vi "RIB Req - eSTOP 1 - Normal Operation.vi"(0 "Limits File Path":path, 5 "Results File Path":path, 11 "error in":errorcluster) -> (4 "Results Data Array":string[][](array[string]), 15 "error out":errorcluster)   [LabVIEW 2024]
doc: "Template test"
uses:
  <vilib>/addons/_JKI Toolkits/State Machine/_JKI_lib_State_Machine.llb/Select State(s)_err__jki_lib_state_machine.vi
  <vilib>/addons/_JKI Toolkits/State Machine/_JKI_lib_State_Machine.llb/Periodic Trigger__ogtk__JKI-SM__jki_lib_state_machine.vi
  <userlib>/_OpenG.lib/file/file.llb/Strip Path Extension - String__ogtk.vi
  <vilib>/Utility/file.llb/Read Delimited Spreadsheet (string).vi
  <vilib>/addons/_JKI Toolkits/State Machine/_JKI_lib_State_Machine.llb/Select State(s)_bool__jki_lib_state_machine.vi
  <userlib>/_OpenG.lib/file/file.llb/openg_file.lvlib
  <userlib>/_OpenG.lib/appcontrol/appcontrol.llb/openg_application_control.lvlib
  <userlib>/_OpenG.lib/time/time.llb/openg_time.lvlib
  <vilib>/Utility/file.llb/Write Delimited Spreadsheet (string).vi
panel:
  out "Timeout - Error Test 2":dbl(slide) scale=0.0..3.0
  out "Wait - Reset":u32(slide)=1 scale=0.0..10.0
  in  "eSTOP 1 State Error Test":string
  in  "eSTOP 1 State Test":string
  in  "Read Start":string
  in  "Read Set":string
  out "Timeout - Error Test":dbl(slide) scale=0.0..3.0
  in  "eSTOP 1 Error Test":string
  in  "eSTOP 1 Test":string
  in  "connection ID":refnum<k16>
  in  "handle out":u64
  in  "Exit":bool
  # "eSTOP 1 Test"
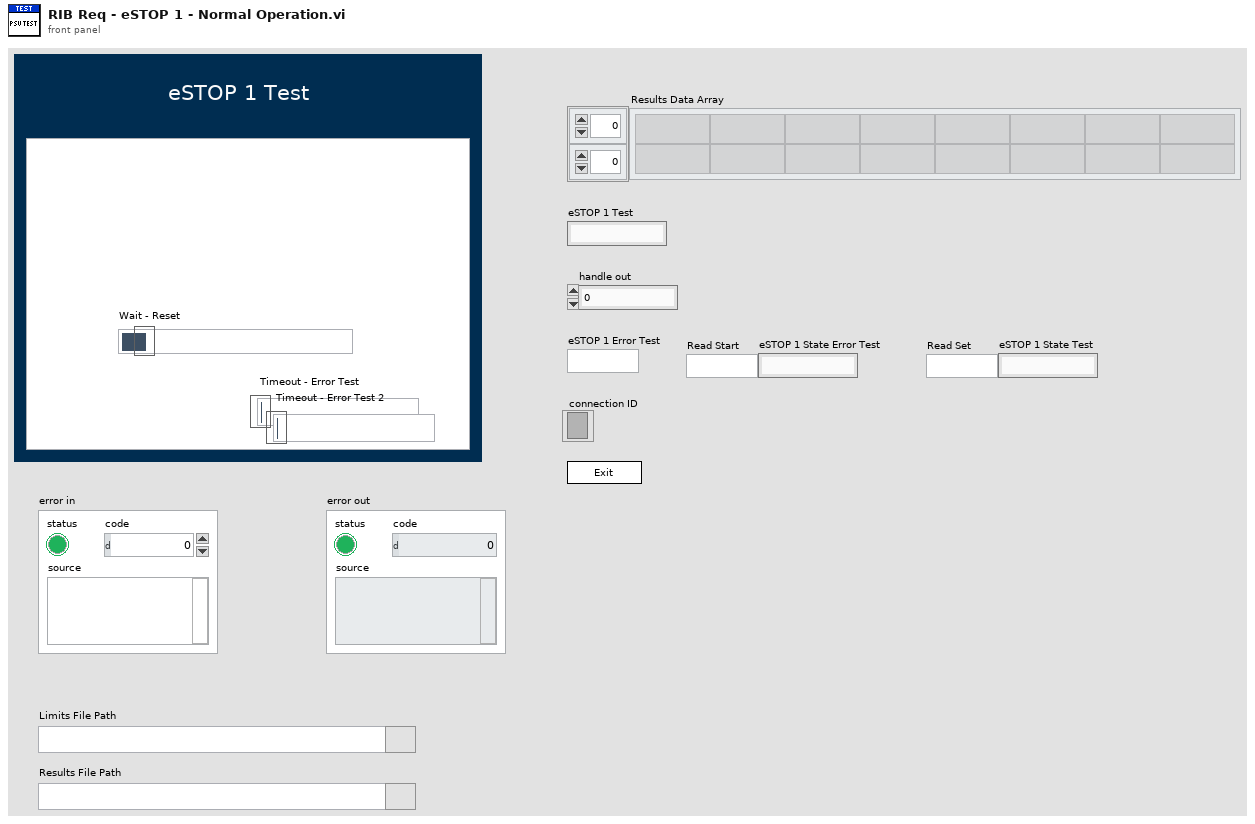
[diagram p1: front panel]
types:
  T1 = enum32{"Invalid", "Standard", "Closed", "Hidden", "Minimized", "Maximized"}
  T2 = enum32{"invalid app kind", "Development System", "Run Time System", "Student Edition", "Embedded LabVIEW", "Evaluation", "Custom"}
  T3 = typedef "FGV - Enum" = enum16{"Cleanup", "Get Data", "Open UDP", "Initialise DAQ", "Initialise I2C"}
  T4 = enum16{"Start Timer", "Get Time", "Pause", "Unpause"}
  T5 = cluster{"Core":cluster{"Current VI Reference":refnum<vi>, "Close Panel on Exit?":bool}, "Limits File Path":path, "Test Limits":string[][], "Results Data Array":string[][], "Results File Path":path, "Voltage":dbl, "connection ID":refnum<k16>, "handle out":u64, "eSTOP 1 Test":string, "eSTOP 1 Error Test":string, "Read Set":string, "Read Start ":string, "eSTOP 1 State Test":string, "eSTOP 1 State Error Test":string}
  T6 = cluster{"Current VI Reference":refnum<vi>, "Close Panel on Exit?":bool}
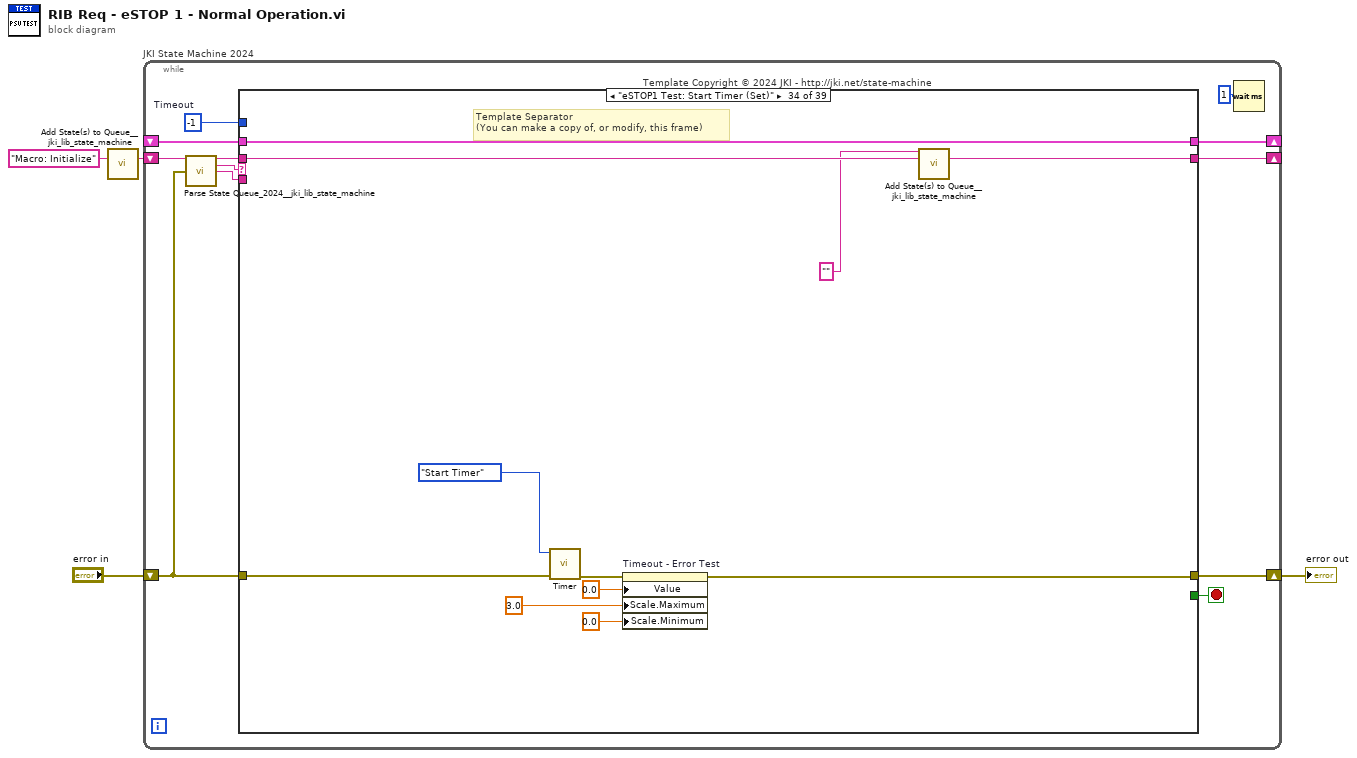
[diagram p0: block diagram]
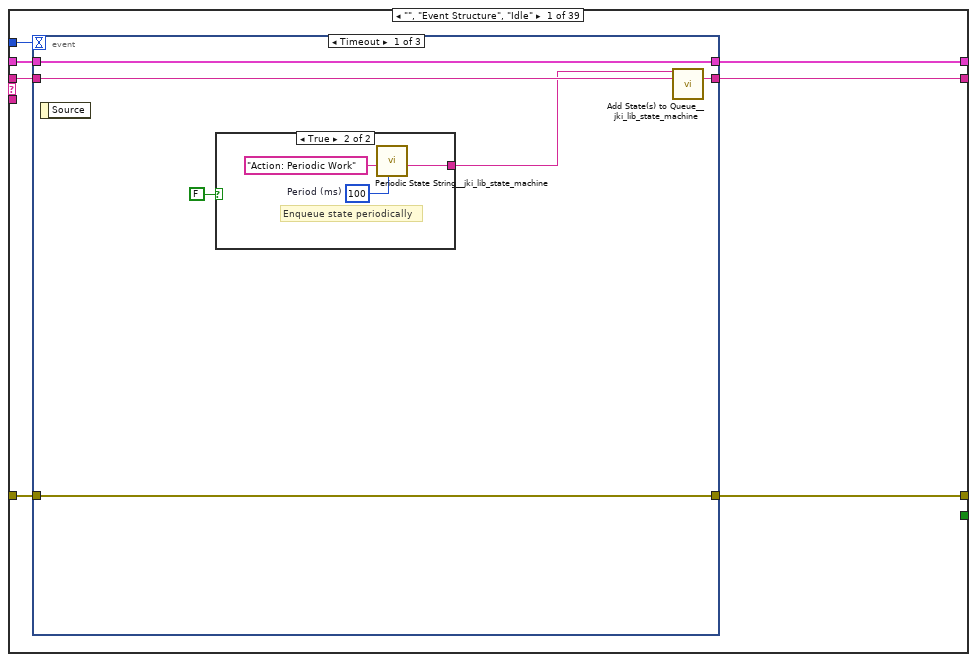
[diagram p2: hidden frame]
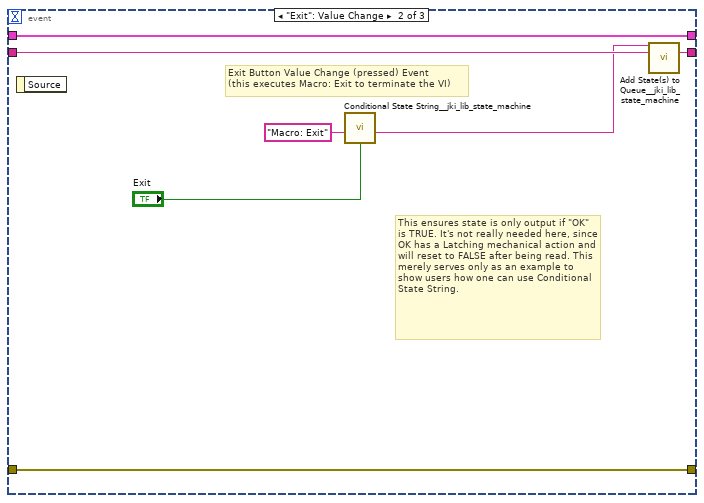
[diagram p4: hidden frame]
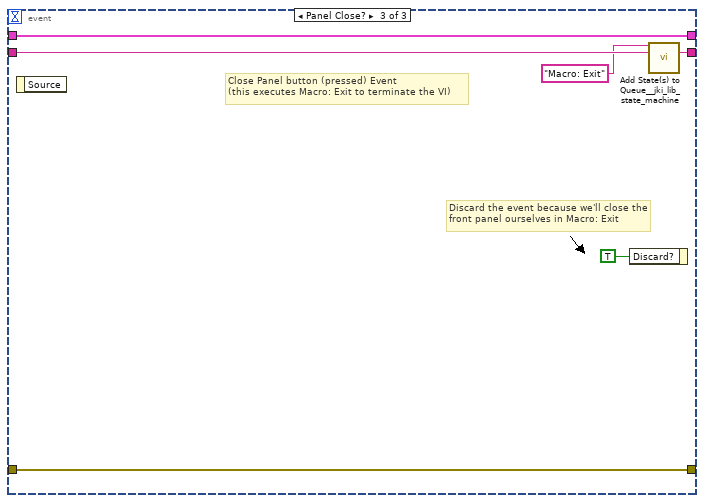
[diagram p5: hidden frame]
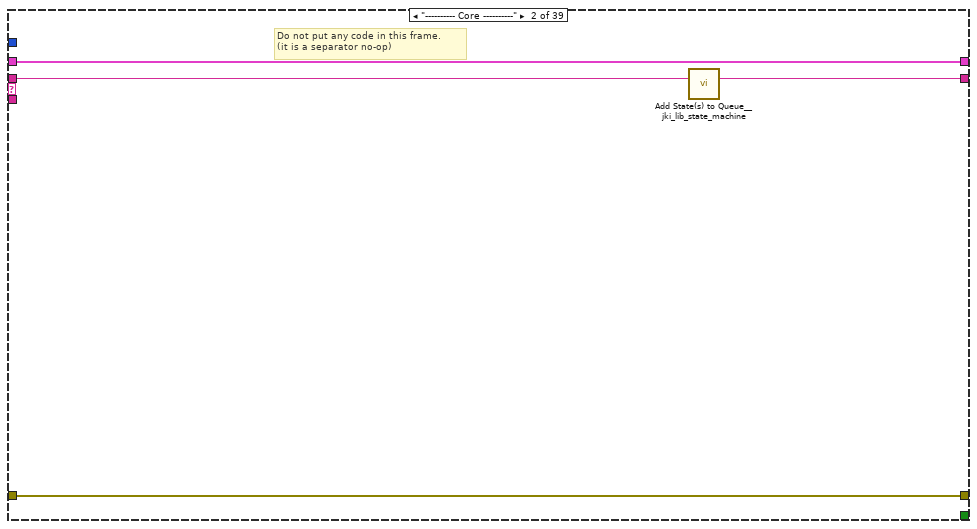
[diagram p6: hidden frame]
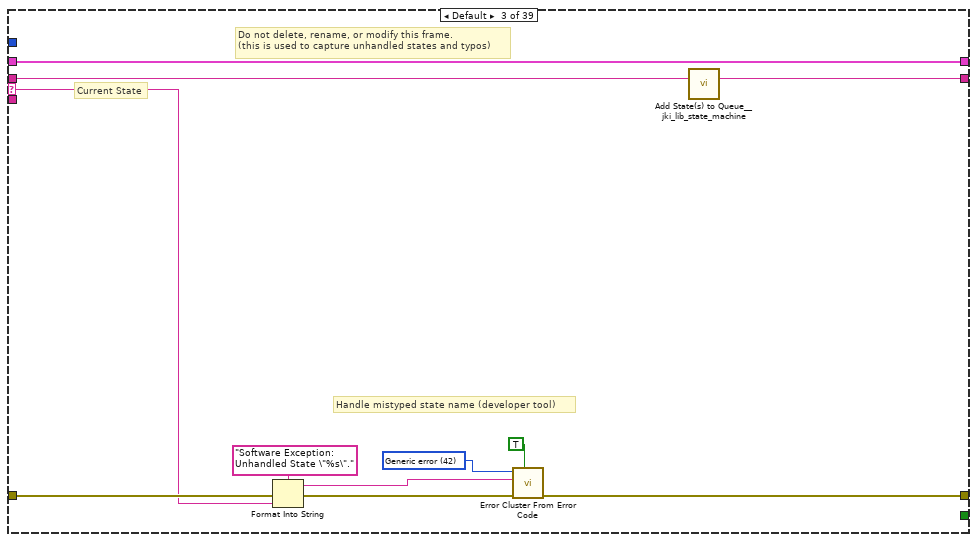
[diagram p7: hidden frame]
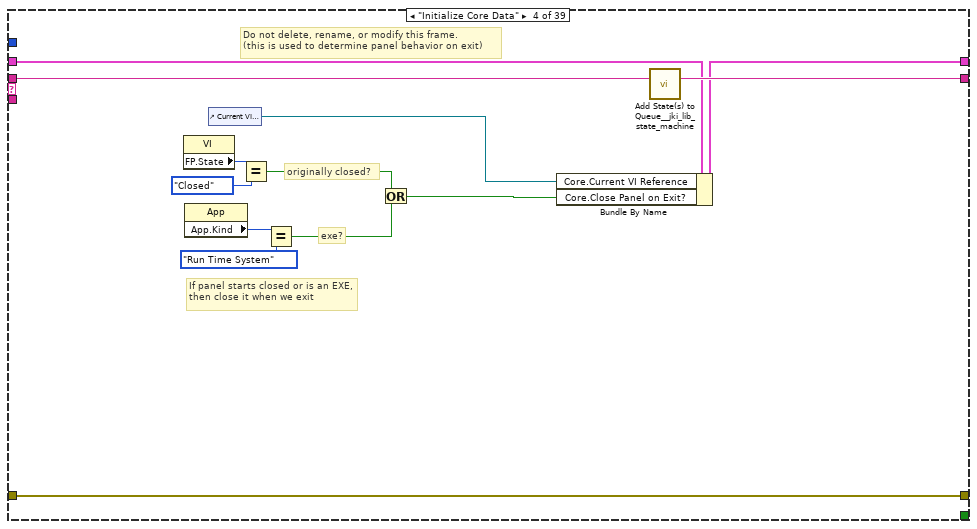
[diagram p8: hidden frame]
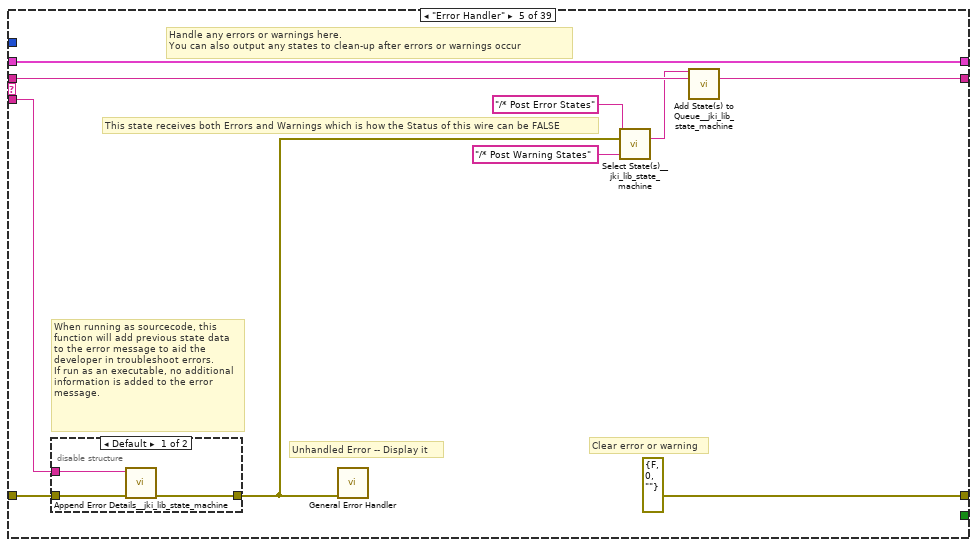
[diagram p9: hidden frame]
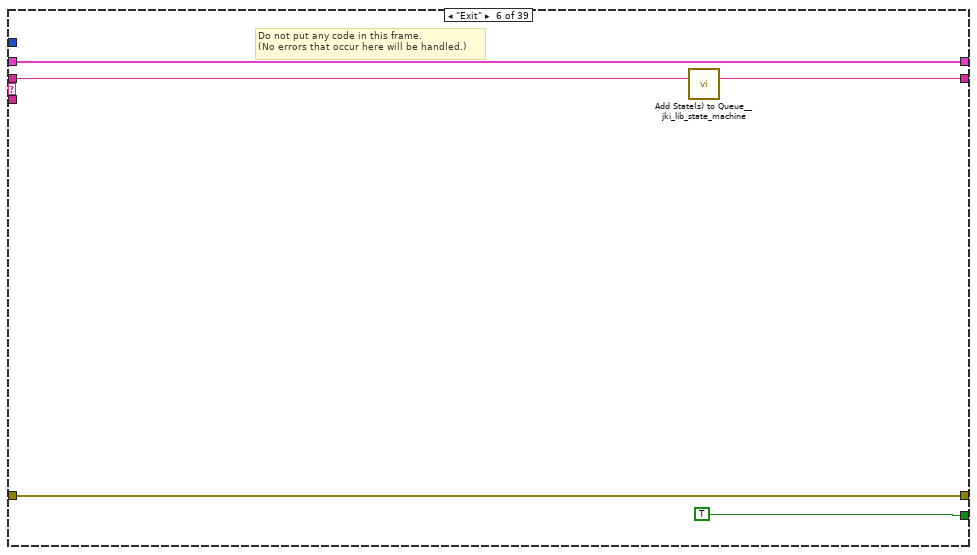
[diagram p11: hidden frame]
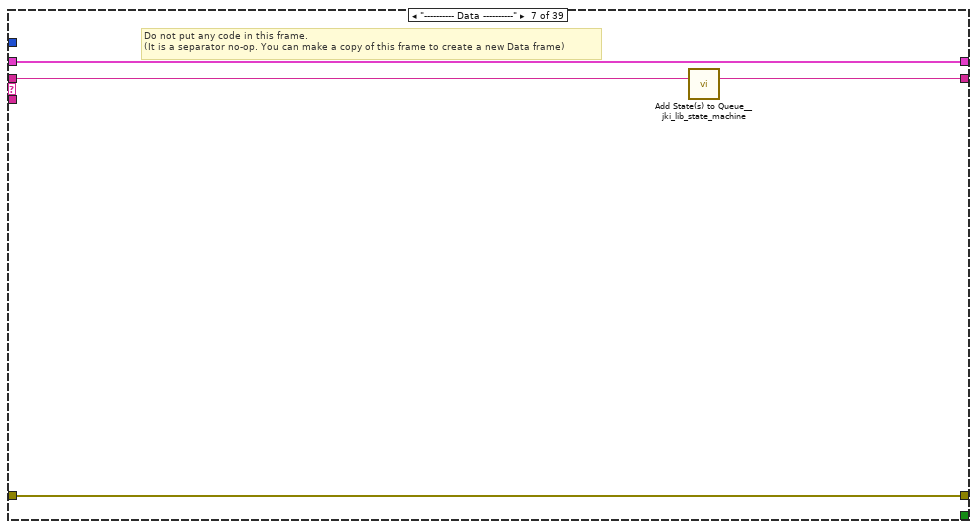
[diagram p12: hidden frame]
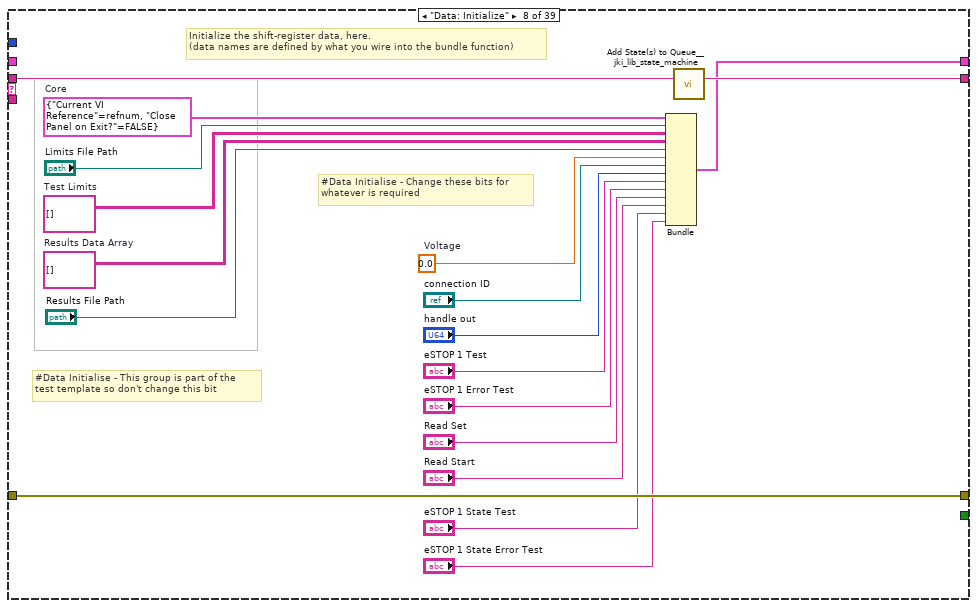
[diagram p13: hidden frame]
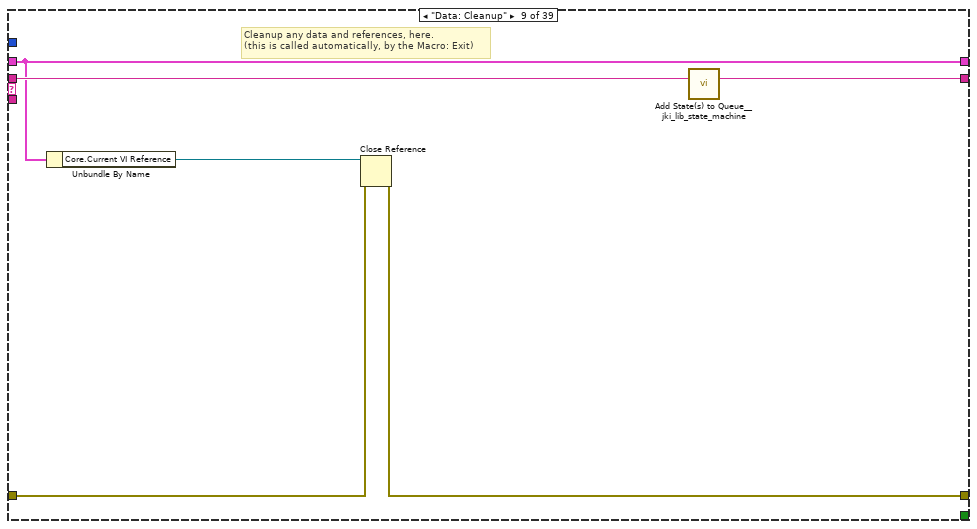
[diagram p14: hidden frame]
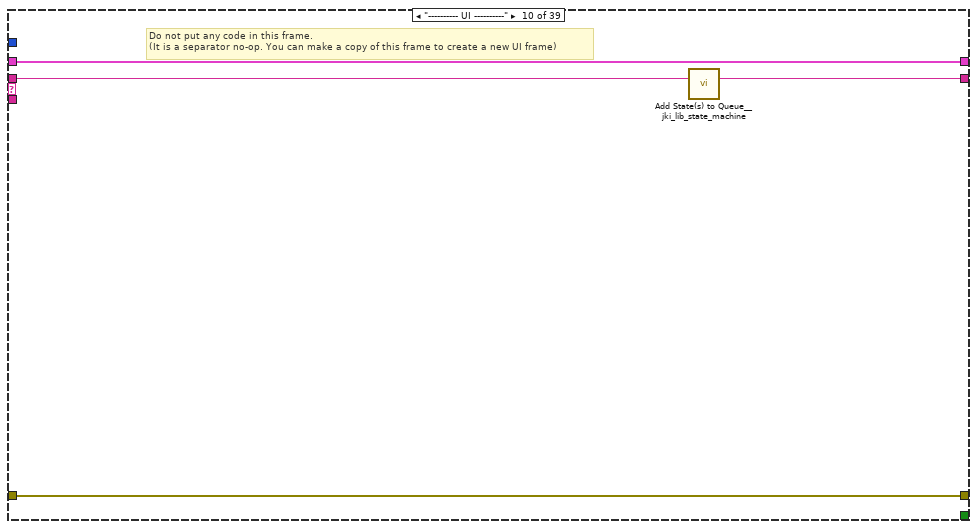
[diagram p15: hidden frame]
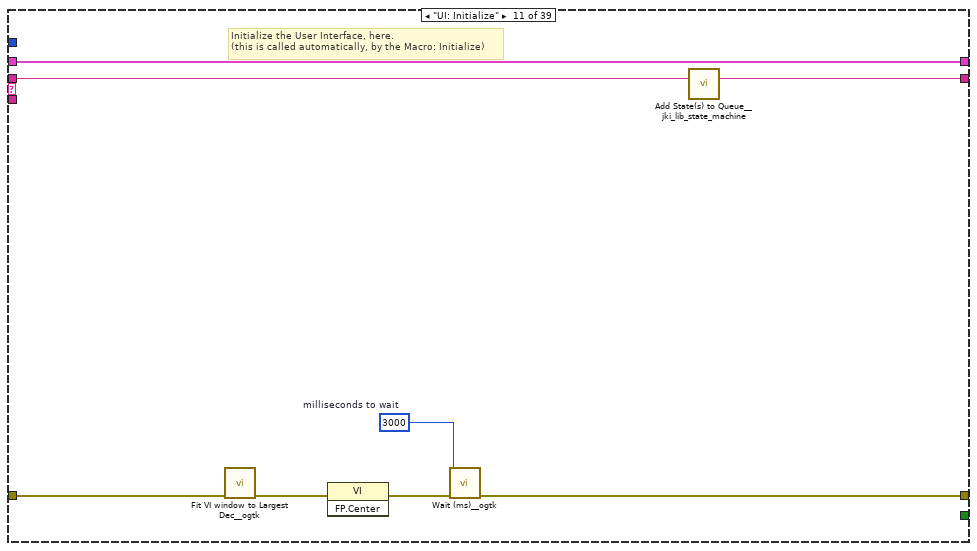
[diagram p16: hidden frame]
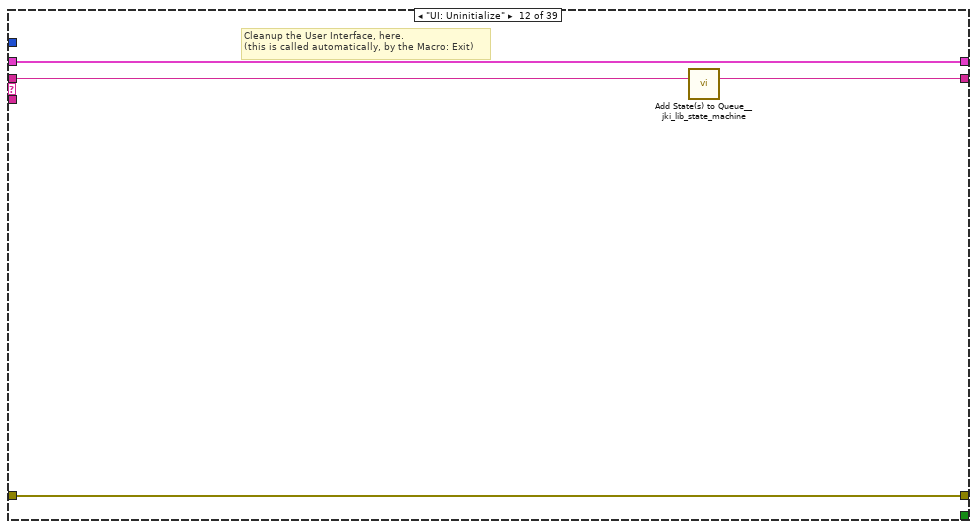
[diagram p17: hidden frame]
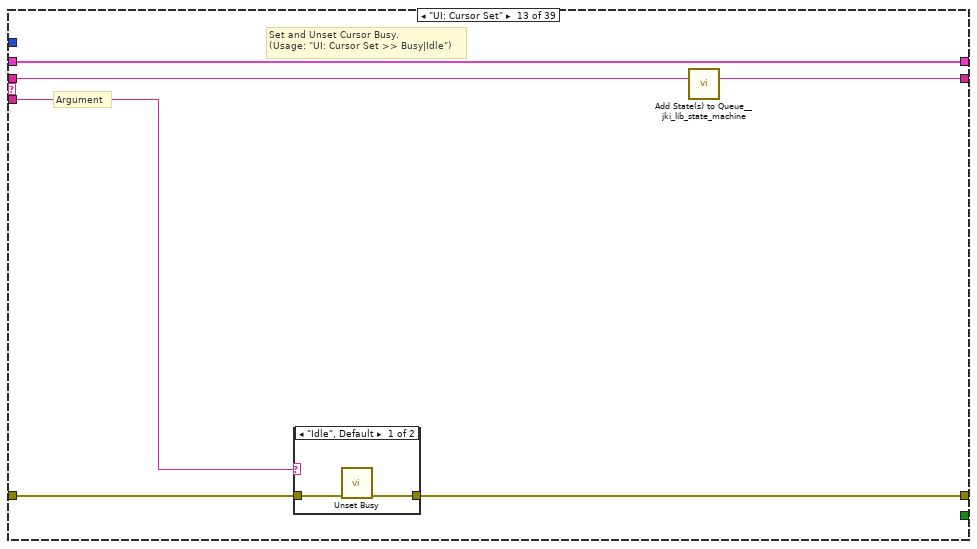
[diagram p18: hidden frame]
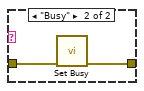
[diagram p19: hidden frame]
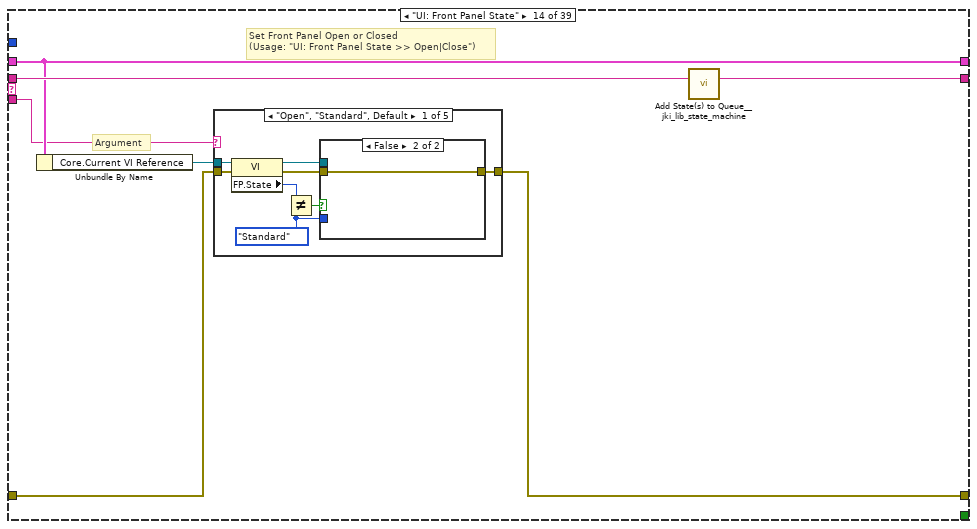
[diagram p20: hidden frame]
diagram:
  n1 = call <vilib>:"Add State(s) to Queue__jki_lib_state_machine.vi"("State(s) in (\"\")"="Macro: Initialize") -> ("States Out"=w4:string)  [unwired: 14 in]
  n2 = while "JKI State Machine 2024" {
    shift-right: [w9] -> _
    shift-left: _ -> [w8]
    shift-right: [w12] -> w1
    shift-left: "error in" -> [w6]
    shift-right: [w11] -> _
    shift-left: w4 -> [w13]
    stop <- w10 stop-if-true
    w7 = -1  # Timeout
    # "Template Copyright © 2024 JKI - http://jki.net/state-machine"
    n3 = call <vilib>:"Parse State Queue_2024__jki_lib_state_machine.vi"("State Queue"=w13, "Error In (no error)"=w6) -> ("Remaining States"=w15:string, "Current State"=w16:string, "Arguments"=w14:string)  [unwired: 11 in]
    n4 = case shown="\"eSTOP1 Test: Start Timer (Set)\"" w16 {
      selector: w16 -> [_ _ w50 _ _ _ _ _ _ _ _ _ _ _ _ _ _ _ _ _ _ _ _ _ _ _ _ _ _ _ _ _ _ _ _ _ _ _ _]
      tunnel: w15 -> [w23 w49 w54 w73 w83 w92 w96 w114 w120 w124 w132 w136 w142 w153 w222 w227 w232 w237 w242 w251 w255 w268 w285 w298 w311 w324 w337 w350 w354 w363 w367 w376 w385 w396 w418 w430 w441 w462 w474]
      tunnel: w14 -> [_ _ _ _ w78 _ _ _ _ _ _ _ w137 w147 _ _ _ _ _ _ _ _ _ _ _ _ _ _ _ _ _ _ _ _ _ _ _ _ _]
      tunnel: w8 -> [w21 w46 w52 w66 w80 w90 w93 _ w115 w121 w130 w134 w140 w149 w219 w224 w229 w234 w239 w249 w252 w258 w277 w290 w303 w316 w329 w342 w351 w359 w364 w374 w378 w394 w415 w428 w439 w459 w472]
      tunnel: [w20 w47 w56 w70 errorcluster {"status"=FALSE, "code"=0, "source"=""} ("error out") w89 w94 w111 w116 w122 w128 w133 w138 w150 w220 w225 w230 w235 w240 w246 w253 w264 w282 w295 w308 w321 w334 w347 w352 w361 w365 w371 w380 w387 w399 w422 w432 w443 w466] -> w12
      tunnel: w6 -> [w17 w47 w55 w70 w79 w89 w94 w111 w117 w122 w129 w133 w139 w151 w220 w225 w230 w235 w240 w246 w253 w263 w281 w294 w307 w320 w333 w346 w352 w360 w365 w372 w379 w388 w414 w423 w433 w458 w467]
      tunnel: [w22 w48 w53 w72 w82 w91 w95 w113 w119 w123 w131 w135 w141 w152 w221 w226 w231 w236 w241 w250 w254 w267 w284 w297 w310 w323 w336 w349 w353 w362 w366 w375 w384 w395 w417 w429 w440 w461 w473] -> w11
      tunnel: [_ _ _ _ _ TRUE _ _ _ _ _ _ _ _ _ _ _ _ _ _ _ _ _ _ _ _ _ _ _ _ _ _ _ _ _ _ _ _ _] -> w10
      tunnel: [w19 w46 w52 w71 w80 w90 w93 w112 w115 w121 w130 w134 w140 w149 w219 w224 w229 w234 w239 w249 w252 w257 w276 w289 w302 w315 w328 w341 w351 w359 w364 w373 w377 w394 w416 w428 w439 w460 w472] -> w9
      tunnel: w7 -> [w18 _ _ _ _ _ _ _ _ _ _ _ _ _ _ _ _ _ _ _ _ _ _ _ _ _ _ _ _ _ _ _ _ _ _ _ _ _ _]
      frame "", "Event Structure", "Idle" {
        n5 = event shown="[0] Timeout" {
          selector: _ -> [_ _ _]
          dyn-events: _ -> [_ _ _]
          timeout: w18 -> [_ _ _]
          tunnel: w23 -> [w29 w39 w45]
          tunnel: [w28 w38 w44] -> w22
          tunnel: w21 -> [w26 w36 w42]
          tunnel: [w27 w37 w43] -> w20
          tunnel: w17 -> [w27 w37 w43]
          tunnel: [w26 w36 w42] -> w19
          event Timeout {
            n6 = event-data() -> ()  [unwired: 1 in, 1 out]
            n7 = case shown="True" FALSE {
              tunnel: [_ w32] -> w25
              frame False {
              }
              frame True {
                w30 = u32 100  # Period (ms)
                # "Enqueue state periodically"
                n8 = call <vilib>:"Periodic State String__jki_lib_state_machine.vi"("Period (ms)"=w30, "State"="Action: Periodic Work") -> ("State Out"=w32:string)  [unwired: 9 in]
              }
            }
            n9 = call <vilib>:"Add State(s) to Queue__jki_lib_state_machine.vi"("State(s) in Front (\"\")"=w25, "State(s) in (\"\")"=w29) -> ("States Out"=w28:string)  [unwired: 13 in]
          }
          event "Exit": Value Change {
            # "This ensures state is only output if \"OK\" is TRUE. It's not really needed here, since OK has a Latching mechanical action and will reset to FALSE after being read. This merely serves only as an example to show users how one can use Conditional State String."
            # "Exit Button Value Change (pressed) Event\n(this executes Macro: Exit to terminate the VI)"
            n10 = event-data() -> ()  [unwired: 1 in, 1 out]
            n11 = call <vilib>:"Conditional State String__jki_lib_state_machine.vi"("Do State(s)?"="Exit", "State"="Macro: Exit") -> ("State Out"=w33:string)  [unwired: 7 in]
            n12 = call <vilib>:"Add State(s) to Queue__jki_lib_state_machine.vi"("State(s) in Front (\"\")"=w33, "State(s) in (\"\")"=w39) -> ("States Out"=w38:string)  [unwired: 13 in]
          }
          event Panel Close? {
            # "Discard the event because we'll close the front panel ourselves in Macro: Exit"
            # "Close Panel button (pressed) Event\n(this executes Macro: Exit to terminate the VI)"
            n13 = event-data() -> ()  [unwired: 1 in, 1 out]
            n14 = event-data("Discard?"=TRUE) -> ()  [unwired: 1 in, 1 out]
            n15 = call <vilib>:"Add State(s) to Queue__jki_lib_state_machine.vi"("State(s) in Front (\"\")"="Macro: Exit", "State(s) in (\"\")"=w45) -> ("States Out"=w44:string)  [unwired: 13 in]
          }
        }
      }
      frame "---------- Core ----------" {
        # "Do not put any code in this frame.\n(it is a separator no-op)"
        n16 = call <vilib>:"Add State(s) to Queue__jki_lib_state_machine.vi"("State(s) in (\"\")"=w49) -> ("States Out"=w48:string)  [unwired: 14 in]
      }
      frame Default {
        w59 = 42 items=["No error", "Argument error", "Memory is full", "Out of zone", "End of file", "File already open", "Generic file I/O error", "File not found", "File permission error", "Disk is full", "Duplicate path", "Too many files open", "System feature not enabled", "Resource file not found", "Cannot add resource", "Resource not found", "Image not found", "Image memory error", "Pen does not exist", "Config type invalid", "Config token not found", "Config parse error", "Config memory error", "Bad external code format", "Bad external code offset", "External code not present", "Null window", "Destroy window error", "Null menu", "Print aborted", "Bad print record", "Print driver error", "Windows error during printing", "Memory error during printing", "Print dialog error", "Generic print error", "Invalid device refnum", "Device not found", "Device parameter error", "Device unit error", "Cannot open device", "Device call aborted", "Generic error", "Cancelled by user", "Object ID too low", "Object ID too high", "Object not in heap", "Unknown heap", "Unknown object (invalid DefProc)", "Unknown object (DefProc not in table)", "Message out of range", "Invalid (null) method", "Unknown message", "Manager call not supported", "Bad address", "Network operation in progress", "Network operation timed out", "Connection is busy", "Network attribute not supported", "Network error", "Address in use", "System out of memory", "Connection aborted", "Connection refused", "Not connected", "Already connected", "Connection closed", "Initialization error (interapplication manager)", "Bad occurrence", "Wait on unbound occurrence handler", "Occurrence queue overflow", "Datalog type conflict", "Unused", "Unrecognized type (interapplication manager)", "Memory corrupt", "Failed to make temporary DLL", "Old CIN version", "Drag socket not found", "Failed to load drop-object", "Failed to register OLE object", "Failed to release OLE object", "Format specifier type mismatch", "Unknown format specifier", "Too few format specifiers", "Too many format specifiers", "Scan failed", "Newer CIN version", "Error converting to variant", "Runtime menu error", "Password tampered", "Variant attribute not found", "Incompatible variant data type", "Event data is not available", "Event Store is not present", "Occurrence is not found", "Event Queue is not created", "Event info is not available", "Refnum passed is NULL", "Error retrieving Class GUID", "Error retrieving CoClass GUID", "Error retrieving TypeLib GUID.", "Bad built application magic bytes.", "Specific driver is different from the specific driver associated with the Logical Name.", "There is no session opened to the class driver.", "Max Error", "MAX - Error with config objects", "MAX - Error loading configuration", "MAX - Group not supported"]
        # "Current State"
        # "Do not delete, rename, or modify this frame.\n(this is used to capture unhandled states and typos)"
        # "Handle mistyped state name (developer tool)"
        n17 = Format Into String(format string="Software Exception: Unhandled State \"%s\"." ("message"), error in=w55, w50) -> (resulting string=w58:string, error out=w57:errorcluster)  [unwired: 1 in]
        n18 = call <vilib>:"Error Cluster From Error Code.vi"("show call chain? (False)"=TRUE, "error in (no error)"=w57, "error message (\"\")"=w58, "error code (0)"=w59) -> ("error out"=w56:errorcluster)  [unwired: 5 in]
        n19 = call <vilib>:"Add State(s) to Queue__jki_lib_state_machine.vi"("State(s) in (\"\")"=w54) -> ("States Out"=w53:string)  [unwired: 14 in]
      }
      frame "Initialize Core Data" {
        # "Do not delete, rename, or modify this frame.\n(this is used to determine panel behavior on exit)"
        # "originally closed?"
        # "exe?"
        # "If panel starts closed or is an EXE, then close it when we exit"
        n20 = property class="VI"() -> ("FP.State"=w63:T1)  [unwired: 2 in, 2 out]
        n21 = property class="App"() -> ("App.Kind"=w69:T2)  [unwired: 2 in, 2 out]
        n22 = control-ref of="Current VI Reference"() -> (w64:refnum<vi>)
        n23 = Equal?(x=w63, y=T1."Closed" ("Front Panel Window:State")) -> (x = y?=w61:bool)
        n24 = Equal?(x=w69, y=T2."Run Time System" ("Application:Kind")) -> (x = y?=w67:bool)
        n25 = Or(x=w61, y=w67) -> (x .or. y?=w65:bool)
        n26 = Bundle By Name(cluster=w66, "Core.Current VI Reference"=w64, "Core.Close Panel on Exit?"=w65) -> (w71:T5)
        n27 = call <vilib>:"Add State(s) to Queue__jki_lib_state_machine.vi"("State(s) in (\"\")"=w73) -> ("States Out"=w72:string)  [unwired: 14 in]
      }
      frame "Error Handler" {
        # "When running as sourcecode, this function will add previous state data to the error message to aid the developer in troubleshoot errors.\nIf run as an executable, no additional information is added to the error message."
        # "This state receives both Errors and Warnings which is how the Status of this wire can be FALSE"
        # "Unhandled Error -- Display it"
        # "Handle any errors or warnings here.\nYou can also output any states to clean-up after errors or warnings occur"
        # "Clear error or warning"
        n28 = disable-structure shown="Default" {
          disable-tunnel: w79 -> [w86 w87]
          disable-tunnel: w78 -> [w85 _]
          disable-tunnel: [w84 w87] -> w77
          frame condition #0 (active) {
            n29 = call <vilib>:"Append Error Details__jki_lib_state_machine.vi"("error in (no error)"=w86, "Previous State and Argument(s)"=w85) -> ("error out"=w84:errorcluster)  [unwired: 9 in]
          }
          frame condition #1 {
          }
        }
        n30 = call <vilib>:"General Error Handler.vi"("error in (no error)"=w77) -> ()  [unwired: 10 in, 5 out]
        n31 = call-poly <vilib>:"Select State(s)__jki_lib_state_machine.vi"("State(s) if True (\"\")"="/* Post Error States", "Select"=w77, "State(s) if False (\"\")"="/* Post Warning States") -> ("States Out"=w75:string)  [unwired: 12 in]
        n32 = call <vilib>:"Add State(s) to Queue__jki_lib_state_machine.vi"("State(s) in Front (\"\")"=w75, "State(s) in (\"\")"=w83) -> ("States Out"=w82:string)  [unwired: 13 in]
      }
      frame "Exit" {
        # "Do not put any code in this frame.\n(No errors that occur here will be handled.)"
        n33 = call <vilib>:"Add State(s) to Queue__jki_lib_state_machine.vi"("State(s) in (\"\")"=w92) -> ("States Out"=w91:string)  [unwired: 14 in]
      }
      frame "---------- Data ----------" {
        # "Do not put any code in this frame.\n(It is a separator no-op. You can make a copy of this frame to create a new Data frame)"
        n34 = call <vilib>:"Add State(s) to Queue__jki_lib_state_machine.vi"("State(s) in (\"\")"=w96) -> ("States Out"=w95:string)  [unwired: 14 in]
      }
      frame "Data: Initialize" {
        w105 = 0.0  # Voltage
        w107 = string[][] []  # Results Data Array
        w108 = string[][] []  # Test Limits
        w110 = T6 {"Current VI Reference"=refnum, "Close Panel on Exit?"=FALSE}  # Core
        # "#Data Initialise - Change these bits for\nwhatever is required"
        # "#Data Initialise - This group is part of the\ntest template so don't change this bit"
        # "Initialize the shift-register data, here.\n(data names are defined by what you wire into the bundle function)"
        n35 = Bundle("Core"=w110, "Limits File Path"="Limits File Path", "Test Limits"=w108, "Results Data Array"=w107, "Results File Path"="Results File Path", "Voltage"=w105, "connection ID"="connection ID", "handle out"="handle out", "eSTOP 1 Test"="eSTOP 1 Test", "eSTOP 1 Error Test"="eSTOP 1 Error Test", "Read Set"="Read Set", "Read Start"="Read Start", "eSTOP 1 State Test"="eSTOP 1 State Test", "eSTOP 1 State Error Test"="eSTOP 1 State Error Test") -> (w112:T5)  [unwired: 1 in]
        n36 = call <vilib>:"Add State(s) to Queue__jki_lib_state_machine.vi"("State(s) in (\"\")"=w114) -> ("States Out"=w113:string)  [unwired: 14 in]
      }
      frame "Data: Cleanup" {
        # "Cleanup any data and references, here.\n(this is called automatically, by the Macro: Exit)"
        n37 = Unbundle By Name(w115) -> ("Core.Current VI Reference"=w118:refnum<vi>)
        n38 = Close Reference(reference=w118, error in (no error)=w117) -> (error out=w116:errorcluster)
        n39 = call <vilib>:"Add State(s) to Queue__jki_lib_state_machine.vi"("State(s) in (\"\")"=w120) -> ("States Out"=w119:string)  [unwired: 14 in]
      }
      frame "---------- UI ----------" {
        # "Do not put any code in this frame.\n(It is a separator no-op. You can make a copy of this frame to create a new UI frame)"
        n40 = call <vilib>:"Add State(s) to Queue__jki_lib_state_machine.vi"("State(s) in (\"\")"=w124) -> ("States Out"=w123:string)  [unwired: 14 in]
      }
      frame "UI: Initialize" {
        w127 = u32 3000  # milliseconds to wait
        # "Initialize the User Interface, here.\n(this is called automatically, by the Macro: Initialize)"
        n41 = call <userlib>:"Fit VI window to Largest Dec__ogtk.vi"("error in (no error)"=w129) -> ("error out"=w125:errorcluster)  [unwired: 5 in, 1 out]
        n42 = invoke class="VI" method="FP.Center"(error in=w125) -> (error out=w126:errorcluster)  [unwired: 2 in, 2 out]
        n43 = call <userlib>:"Wait (ms)__ogtk.vi"("error in (no error)"=w126, "milliseconds to wait"=w127) -> ("error out"=w128:errorcluster)  [unwired: 8 in, 1 out]
        n44 = call <vilib>:"Add State(s) to Queue__jki_lib_state_machine.vi"("State(s) in (\"\")"=w132) -> ("States Out"=w131:string)  [unwired: 14 in]
      }
      frame "UI: Uninitialize" {
        # "Cleanup the User Interface, here.\n(this is called automatically, by the Macro: Exit)"
        n45 = call <vilib>:"Add State(s) to Queue__jki_lib_state_machine.vi"("State(s) in (\"\")"=w136) -> ("States Out"=w135:string)  [unwired: 14 in]
      }
      frame "UI: Cursor Set" {
        # "Argument"
        # "Set and Unset Cursor Busy.\n(Usage: \"UI: Cursor Set >> Busy|Idle\")"
        n46 = case shown="\"Idle\", Default" w137 {
          tunnel: w139 -> [w144 w146]
          tunnel: [w143 w145] -> w138
          frame "Idle", Default {
            n47 = call <vilib>:"Unset Busy.vi"("error in (no error)"=w144) -> ("error out"=w143:errorcluster)  [unwired: 10 in]
          }
          frame "Busy" {
            n48 = call <vilib>:"Set Busy.vi"("error in (no error)"=w146) -> ("error out"=w145:errorcluster)  [unwired: 9 in, 1 out]
          }
        }
        n49 = call <vilib>:"Add State(s) to Queue__jki_lib_state_machine.vi"("State(s) in (\"\")"=w142) -> ("States Out"=w141:string)  [unwired: 14 in]
      }
      frame "UI: Front Panel State" {
        # "Argument"
        # "Set Front Panel Open or Closed\n(Usage: \"UI: Front Panel State >> Open|Close\")"
        n50 = Unbundle By Name(w149) -> ("Core.Current VI Reference"=w148:refnum<vi>)
        n51 = case shown="\"Open\", \"Standard\", Default" w147 {
          tunnel: w151 -> [w159 w174 w185 w198 w211]
          tunnel: [w161 w175 w187 w200 w213] -> w150
          tunnel: w148 -> [w160 w172 w186 w199 w212]
          frame "Open", "Standard", Default {
            w154 = T1."Standard" ("State")
            n52 = property class="VI"(reference=w160, error in=w159) -> (reference out=w157:refnum<vi>, error out=w158:errorcluster, "FP.State"=w156:T1)
            n53 = Not Equal?(x=w156, y=w154) -> (x != y?=w155:bool)
            n54 = case shown="False" w155 {
              tunnel: [w165 w167] -> w161
              tunnel: w158 -> [w164 w167]
              tunnel: w157 -> [w163 _]
              tunnel: w154 -> [w162 _]
              frame True {
                n55 = invoke class="VI" method="FP.Open"(reference=w163, error in=w164, "Activate"=TRUE, "State"=w162) -> (error out=w165:errorcluster)  [unwired: 1 in, 4 out]
              }
              frame False {
              }
            }
          }
          frame "Close", "Closed" {
            n56 = property class="VI"(reference=w172, error in=w174) -> (reference out=w171:refnum<vi>, error out=w173:errorcluster, "FP.State"=w169:T1)
            n57 = Not Equal?(x=w169, y=T1."Closed" ("Front Panel Window:State")) -> (x != y?=w168:bool)
            n58 = case shown="True" w168 {
              tunnel: [w176 w179] -> w175
              tunnel: w173 -> [w176 w178]
              tunnel: w171 -> [_ w177]
              frame False {
              }
              frame True {
                n59 = invoke class="VI" method="FP.Close"(reference=w177, error in=w178) -> (error out=w179:errorcluster)  [unwired: 1 in, 2 out]
              }
            }
          }
          frame "Hidden", "Hide" {
            w180 = T1."Hidden" ("State")
            n60 = property class="VI"(reference=w186, error in=w185) -> (reference out=w183:refnum<vi>, error out=w184:errorcluster, "FP.State"=w182:T1)
            n61 = Not Equal?(x=w182, y=w180) -> (x != y?=w181:bool)
            n62 = case shown="True" w181 {
              tunnel: [w191 w192] -> w187
              tunnel: w184 -> [w190 w192]
              tunnel: w183 -> [w189 _]
              tunnel: w180 -> [w188 _]
              frame True {
                n63 = invoke class="VI" method="FP.Open"(reference=w189, error in=w190, "State"=w188) -> (error out=w191:errorcluster)  [unwired: 2 in, 4 out]
              }
              frame False {
              }
            }
          }
          frame "Minimize", "Minimized" {
            w193 = T1."Minimized" ("State")
            n64 = property class="VI"(reference=w199, error in=w198) -> (reference out=w196:refnum<vi>, error out=w197:errorcluster, "FP.State"=w195:T1)
            n65 = Not Equal?(x=w195, y=w193) -> (x != y?=w194:bool)
            n66 = case shown="True" w194 {
              tunnel: [w204 w205] -> w200
              tunnel: w197 -> [w203 w205]
              tunnel: w196 -> [w202 _]
              tunnel: w193 -> [w201 _]
              frame True {
                n67 = invoke class="VI" method="FP.Open"(reference=w202, error in=w203, "State"=w201) -> (error out=w204:errorcluster)  [unwired: 2 in, 4 out]
              }
              frame False {
              }
            }
          }
          frame "Maximize", "Maximized" {
            w206 = T1."Maximized" ("State")
            n68 = property class="VI"(reference=w212, error in=w211) -> (reference out=w209:refnum<vi>, error out=w210:errorcluster, "FP.State"=w208:T1)
            n69 = Not Equal?(x=w208, y=w206) -> (x != y?=w207:bool)
            n70 = case shown="True" w207 {
              tunnel: [w217 w218] -> w213
              tunnel: w210 -> [w216 w218]
              tunnel: w209 -> [w215 _]
              tunnel: w206 -> [w214 _]
              frame True {
                n71 = invoke class="VI" method="FP.Open"(reference=w215, error in=w216, "State"=w214) -> (error out=w217:errorcluster)  [unwired: 2 in, 4 out]
              }
              frame False {
              }
            }
          }
        }
        n72 = call <vilib>:"Add State(s) to Queue__jki_lib_state_machine.vi"("State(s) in (\"\")"=w153) -> ("States Out"=w152:string)  [unwired: 14 in]
      }
      frame "---------- Macro ----------" {
        # "Do not put any code in this frame.\n(It is a separator no-op. You can make a copy of this frame to create a new Macro frame)"
        n73 = call <vilib>:"Add State(s) to Queue__jki_lib_state_machine.vi"("State(s) in (\"\")"=w222) -> ("States Out"=w221:string)  [unwired: 14 in]
      }
      frame "Macro: Initialize" {
        # "Initialization Macro\n(This is called once, when the VI starts)"
        n74 = call <vilib>:"Add State(s) to Queue__jki_lib_state_machine.vi"("State(s) in Front (\"\")"="Data: Initialize\nInitialize Core Data\nUI: Initialize\nUI: Front Panel State >> Open\neSTOP1 Test: Initialise\nMacro: Test", "State(s) in (\"\")"=w227) -> ("States Out"=w226:string)  [unwired: 13 in]
      }
      frame "Macro: Test" {
        # "#Test Macro - Add the sequence \nfor measurments and limits testing here"
        n75 = call <vilib>:"Add State(s) to Queue__jki_lib_state_machine.vi"("State(s) in Front (\"\")"="Limits Test: Read Limits File\neSTOP1 Test: Initialise", "State(s) in (\"\")"=w232) -> ("States Out"=w231:string)  [unwired: 13 in]
      }
      frame "Macro: Test (Error)" {
        # "#Test Macro - Add the sequence \nfor measurments and limits testing here"
        n76 = call <vilib>:"Add State(s) to Queue__jki_lib_state_machine.vi"("State(s) in Front (\"\")"="eSTOP1 Test: Reset", "State(s) in (\"\")"=w237) -> ("States Out"=w236:string)  [unwired: 13 in]
      }
      frame "Macro: Limits" {
        # "Do not put any code in this frame.\n(It is a separator no-op. You can make a copy of this frame to create a new Macro frame)"
        n77 = call <vilib>:"Add State(s) to Queue__jki_lib_state_machine.vi"("State(s) in Front (\"\")"="Limits Test: eSTOP 1 Test\nLimits Test: eSTOP 1 Error Test\nLimits Test: Read Set\nLimits Test: Read Start\nLimits Test: eSTOP 1 State Error Test\nLimits Test: eSTOP 1 State Test\nResults Data: Write Results Data\nMacro: Exit", "State(s) in (\"\")"=w242) -> ("States Out"=w241:string)  [unwired: 13 in]
      }
      frame "Macro: Exit" {
        # "Exit Macro\n(This is called once, when the VI exits)"
        n78 = Unbundle By Name(w249) -> ("Core.Close Panel on Exit?"=w244:bool)
        n79 = call <vilib>:"Conditional State String__jki_lib_state_machine.vi"("Do State(s)?"=w244, "State"="UI: Front Panel State >> Close") -> ("State Out"=w243:string)  [unwired: 7 in]
        n80 = call <vilib>:"Add State(s) to Queue__jki_lib_state_machine.vi"("State(s) in (\"\")"=w243, "State(s) at Back (\"\")"="UI: Uninitialize\nData: Cleanup\nExit") -> ("States Out"=w247:string)  [unwired: 13 in]
        n81 = call <vilib>:"Add State(s) to Queue__jki_lib_state_machine.vi"("State(s) in Front (\"\")"=w247, "State(s) in (\"\")"=w251) -> ("States Out"=w250:string)  [unwired: 13 in]
      }
      frame "---------- Limits Test ----------" {
        # "Template Separator\n(You can make a copy of, or modify, this frame)"
        n82 = call <vilib>:"Add State(s) to Queue__jki_lib_state_machine.vi"("State(s) in (\"\")"=w255) -> ("States Out"=w254:string)  [unwired: 14 in]
      }
      frame "Limits Test: Read Limits File" {
        w261 = ","  # delimiter (\t)
        n83 = Unbundle By Name(w258) -> ("Limits File Path"=w262:path)
        n84 = Current VI's Path "Test Case Path"() -> (path=w266:path)
        n85 = call-poly <vilib>:"Read Delimited Spreadsheet.vi"("file path (dialog if empty)"=w262, "error in (no error)"=w263, "delimiter (\\t)"=w261) -> ("all rows"=w259:string[][], "error out"=w264:errorcluster)  [unwired: 7 in, 4 out]
        n86 = Strip Path(path=w266) -> (name=w265:string)  [unwired: 1 out]
        n87 = call-poly <userlib>:"Strip Path Extension__ogtk.vi"("path"=w265) -> ("root"=w260:string)  [unwired: 1 out]
        n88 = for {
          tunnel: w260 -> [w272]
          tunnel: w259 -> [w270] mode=indexing
          tunnel: [w270] -> w256 mode=indexing if=w269
          n89 = Index Array(array=w270) -> (element=w271:string)  [unwired: 1 in]
          n90 = Equal?(x=w272, y=w271) -> (x = y?=w269:bool)
        }
        n91 = Bundle By Name(cluster=w258, "Test Limits"=w256) -> (w257:T5)
        n92 = call <vilib>:"Add State(s) to Queue__jki_lib_state_machine.vi"("State(s) in (\"\")"=w268) -> ("States Out"=w267:string)  [unwired: 14 in]
      }
      frame "Limits Test: eSTOP 1 Test" {
        w278 = "eSTOP 1 Test"  # Sub Test Name
        # "Equal to F1?"
        # "#Limits Testing - Add the sub test name for\ntest included in limits file"
        n93 = Unbundle By Name(w277) -> ("Test Limits"=w279:string[][], "eSTOP 1 Test"=w283:string)
        n94 = Unbundle By Name(w277) -> ("Results Data Array"=w275:string[][])
        n95 = To Variant(anything=w283) -> (Variant=w280:variant)
        n96 = call "Process Results.vi"("error in (no error)"=w281, "Measurement"=w280, "Test Limits"=w279, "Sub Test Name"=w278) -> ("error out"=w282:errorcluster, "Results Data"=w274:string[])  [unwired: 6 in]
        n97 = Build Array (concatenate)(w275, w274) -> (w273:string[][])
        n98 = Bundle By Name(cluster=w277, "Results Data Array"=w273) -> (w276:T5)
        n99 = call <vilib>:"Add State(s) to Queue__jki_lib_state_machine.vi"("State(s) in (\"\")"=w285) -> ("States Out"=w284:string)  [unwired: 14 in]
      }
      frame "Limits Test: eSTOP 1 State Test" {
        w291 = "eSTOP 1 State Test"  # Sub Test Name
        # "Equal to F1?"
        # "#Limits Testing - Add the sub test name for\ntest included in limits file"
        n100 = Unbundle By Name(w290) -> ("Test Limits"=w292:string[][], "eSTOP 1 State Test"=w296:string)
        n101 = Unbundle By Name(w290) -> ("Results Data Array"=w288:string[][])
        n102 = To Variant(anything=w296) -> (Variant=w293:variant)
        n103 = call "Process Results.vi"("error in (no error)"=w294, "Measurement"=w293, "Test Limits"=w292, "Sub Test Name"=w291) -> ("error out"=w295:errorcluster, "Results Data"=w287:string[])  [unwired: 6 in]
        n104 = Build Array (concatenate)(w288, w287) -> (w286:string[][])
        n105 = Bundle By Name(cluster=w290, "Results Data Array"=w286) -> (w289:T5)
        n106 = call <vilib>:"Add State(s) to Queue__jki_lib_state_machine.vi"("State(s) in (\"\")"=w298) -> ("States Out"=w297:string)  [unwired: 14 in]
      }
      frame "Limits Test: Read Set" {
        w304 = "Read Set Test"  # Sub Test Name
        # "Equal to F1?"
        # "#Limits Testing - Add the sub test name for\ntest included in limits file"
        n107 = Unbundle By Name(w303) -> ("Results Data Array"=w301:string[][])
        n108 = Unbundle By Name(w303) -> ("Test Limits"=w305:string[][], "Read Set"=w309:string)
        n109 = To Variant(anything=w309) -> (Variant=w306:variant)
        n110 = call "Process Results.vi"("error in (no error)"=w307, "Measurement"=w306, "Test Limits"=w305, "Sub Test Name"=w304) -> ("error out"=w308:errorcluster, "Results Data"=w300:string[])  [unwired: 6 in]
        n111 = Build Array (concatenate)(w301, w300) -> (w299:string[][])
        n112 = Bundle By Name(cluster=w303, "Results Data Array"=w299) -> (w302:T5)
        n113 = call <vilib>:"Add State(s) to Queue__jki_lib_state_machine.vi"("State(s) in (\"\")"=w311) -> ("States Out"=w310:string)  [unwired: 14 in]
      }
      frame "Limits Test: Read Start" {
        w317 = "Read Start Test"  # Sub Test Name
        # "Equal to F1?"
        # "#Limits Testing - Add the sub test name for\ntest included in limits file"
        n114 = Unbundle By Name(w316) -> ("Results Data Array"=w314:string[][])
        n115 = Unbundle By Name(w316) -> ("Test Limits"=w318:string[][], "Read Start"=w322:string)
        n116 = To Variant(anything=w322) -> (Variant=w319:variant)
        n117 = call "Process Results.vi"("error in (no error)"=w320, "Measurement"=w319, "Test Limits"=w318, "Sub Test Name"=w317) -> ("error out"=w321:errorcluster, "Results Data"=w313:string[])  [unwired: 6 in]
        n118 = Build Array (concatenate)(w314, w313) -> (w312:string[][])
        n119 = Bundle By Name(cluster=w316, "Results Data Array"=w312) -> (w315:T5)
        n120 = call <vilib>:"Add State(s) to Queue__jki_lib_state_machine.vi"("State(s) in (\"\")"=w324) -> ("States Out"=w323:string)  [unwired: 14 in]
      }
      frame "Limits Test: eSTOP 1 Error Test" {
        w330 = "eSTOP 1 Error Test"  # Sub Test Name
        # "Equal to FF ?"
        # "#Limits Testing - Add the sub test name for\ntest included in limits file"
        n121 = Unbundle By Name(w329) -> ("Test Limits"=w331:string[][], "eSTOP 1 Error Test"=w335:string)
        n122 = Unbundle By Name(w329) -> ("Results Data Array"=w327:string[][])
        n123 = To Variant(anything=w335) -> (Variant=w332:variant)
        n124 = call "Process Results.vi"("error in (no error)"=w333, "Measurement"=w332, "Test Limits"=w331, "Sub Test Name"=w330) -> ("error out"=w334:errorcluster, "Results Data"=w326:string[])  [unwired: 6 in]
        n125 = Build Array (concatenate)(w327, w326) -> (w325:string[][])
        n126 = Bundle By Name(cluster=w329, "Results Data Array"=w325) -> (w328:T5)
        n127 = call <vilib>:"Add State(s) to Queue__jki_lib_state_machine.vi"("State(s) in (\"\")"=w337) -> ("States Out"=w336:string)  [unwired: 14 in]
      }
      frame "Limits Test: eSTOP 1 State Error Test" {
        w343 = "eSTOP 1 State Error Test"  # Sub Test Name
        # "Equal to FF ?"
        # "#Limits Testing - Add the sub test name for\ntest included in limits file"
        n128 = Unbundle By Name(w342) -> ("Test Limits"=w344:string[][], "eSTOP 1 State Error Test"=w348:string)
        n129 = Unbundle By Name(w342) -> ("Results Data Array"=w340:string[][])
        n130 = To Variant(anything=w348) -> (Variant=w345:variant)
        n131 = call "Process Results.vi"("error in (no error)"=w346, "Measurement"=w345, "Test Limits"=w344, "Sub Test Name"=w343) -> ("error out"=w347:errorcluster, "Results Data"=w339:string[])  [unwired: 6 in]
        n132 = Build Array (concatenate)(w340, w339) -> (w338:string[][])
        n133 = Bundle By Name(cluster=w342, "Results Data Array"=w338) -> (w341:T5)
        n134 = call <vilib>:"Add State(s) to Queue__jki_lib_state_machine.vi"("State(s) in (\"\")"=w350) -> ("States Out"=w349:string)  [unwired: 14 in]
      }
      frame "---------- Results Data ----------" {
        # "Template Separator\n(You can make a copy of, or modify, this frame)"
        n135 = call <vilib>:"Add State(s) to Queue__jki_lib_state_machine.vi"("State(s) in (\"\")"=w354) -> ("States Out"=w353:string)  [unwired: 14 in]
      }
      frame "Results Data: Write Results Data" {
        w356 = ","  # delimiter (\t)
        w357 = TRUE  # append to file? (new file:F)
        n136 = Unbundle By Name(w359) -> ("Results File Path"=w358:path, "Results Data Array"=w355:string[][])
        "Results Data Array" <- w355
        n137 = call-poly <vilib>:"Write Delimited Spreadsheet.vi"("file path (dialog if empty)"=w358, "2D data"=w355, "append to file? (new file:F)"=w357, "error in (no error)"=w360, "delimiter (\\t)"=w356) -> ("error out"=w361:errorcluster)  [unwired: 9 in, 1 out]
        n138 = call <vilib>:"Add State(s) to Queue__jki_lib_state_machine.vi"("State(s) in (\"\")"=w363) -> ("States Out"=w362:string)  [unwired: 14 in]
      }
      frame "---------- eSTOP1 Test ----------" {
        # "Template Separator\n(You can make a copy of, or modify, this frame)"
        n139 = call <vilib>:"Add State(s) to Queue__jki_lib_state_machine.vi"("State(s) in (\"\")"=w367) -> ("States Out"=w366:string)  [unwired: 14 in]
      }
      frame "eSTOP1 Test: Initialise" {
        # "Measurement initialisation code goes here"
        n140 = call "FGV - Initialise.vi"("Enum"=FGV_-_Enum."Get Data", "Error In"=w372) -> ("connection ID"=w369:refnum<k16>, "Handle Out"=w368:u64, "Error Out"=w371:errorcluster)  [unwired: 10 in, 1 out]
        n141 = Bundle By Name(cluster=w374, "connection ID"=w369, "handle out"=w368) -> (w373:T5)
        n142 = call <vilib>:"Add State(s) to Queue__jki_lib_state_machine.vi"("State(s) in (\"\")"=w376) -> ("States Out"=w375:string)  [unwired: 14 in]
      }
      frame "eSTOP1 Test: Reset" {
        # "Switch relays - back to Initialize state"
        # "Measurment cleanup code goes here"
        n143 = Unbundle By Name(w378) -> ("handle out"=w382:u64)
        n144 = call "PCA9525 - Estop 1.vi"("error in (no error)"=w379, "buffer"=u8[] [2, 85, 0], "handle"=w382) -> ("error out"=w380:errorcluster, "handle out"=w381:u64)  [unwired: 6 in, 1 out]
        n145 = Bundle By Name(cluster=w378, "handle out"=w381) -> (w377:T5)
        n146 = call <vilib>:"Add State(s) to Queue__jki_lib_state_machine.vi"("State(s) in (\"\")"=w385) -> ("States Out"=w384:string)  [unwired: 14 in]
      }
      frame "eSTOP1 Test: Start Timer (Set)" {
        # "Template Separator\n(You can make a copy of, or modify, this frame)"
        n147 = call "Timer.vi"("error in (no error)"=w388, "Enum"=T4."Start Timer") -> ("error out"=w392:errorcluster)  [unwired: 6 in, 3 out]
        n148 = property on="Timeout - Error Test" class="Slide (strict)"(error in=w392, "Value"=0.0 ("Horizontal Pointer Slide"), "Scale.Maximum"=3.0 ("Target Time"), "Scale.Minimum"=0.0 ("Scale.Range:Minimum")) -> (error out=w387:errorcluster)  [unwired: 1 in, 1 out]
        n149 = call <vilib>:"Add State(s) to Queue__jki_lib_state_machine.vi"("State(s) in Front (\"\")"="" ("State(s) if True (\"\")"), "State(s) in (\"\")"=w396) -> ("States Out"=w395:string)  [unwired: 13 in]
      }
      frame "eSTOP1 Test: Set Command (Error)" {
        # "Data"
        # "Length"
        # "ID"
        # "Target"
        # "Type"
        # "Pkt ID"
        # "Measurement initialisation code goes here"
        n150 = Unbundle By Name(w415) -> ("connection ID"=w413:refnum<k16>)
        n151 = Build Array(u8 91 ("element"), u8 1 ("element"), u8 9 ("element"), u8 108 ("element"), u8 0 ("element")) -> (w407:u8[])
        n152 = String To IP(1:"192.168.201.21" ("name")) -> (0:w411:u32)
        n153 = Byte Array To String(unsigned byte array=w407) -> (string=w401:string)
        n154 = UDP Write(address=w411, port or service name=u16 54321, connection ID=w413, data in=w401, 8:w414, 9:1000 ("timeout ms (25000)")) -> (error out=w400:errorcluster, 3:w412:refnum<k16>)
        n155 = Bundle By Name(cluster=w415, "connection ID"=w412) -> (w416:T5)
        n156 = call <userlib>:"Wait (ms)__ogtk.vi"("error in (no error)"=w400, "milliseconds to wait"=u32 20000) -> ("error out"=w399:errorcluster, "millisecond timer value"=→"Wait - Reset":u32)  [unwired: 8 in]
        n157 = call <vilib>:"Add State(s) to Queue__jki_lib_state_machine.vi"("State(s) in (\"\")"=w418) -> ("States Out"=w417:string)  [unwired: 14 in]
      }
      frame "eSTOP1 Test: Elapsed Timer (Set)" {
        # "check if timer elapsed if true end of test if false UDP is read again,"
        # "Template Separator\n(You can make a copy of, or modify, this frame)"
        n158 = call "Timer.vi"("error in (no error)"=w423, "Target Time"=3.0, "Enum"=T4."Get Time") -> ("error out"=w422:errorcluster, "Time Elapsed?"=w424:bool, "Elapsed Time"=→"Timeout - Error Test":dbl)  [unwired: 5 in, 1 out]
        n159 = call-poly <vilib>:"Select State(s)__jki_lib_state_machine.vi"("State(s) if True (\"\")"="Macro: Limits" ("State(s) if True (\"\")"), "Select"=w424, "State(s) if False (\"\")"="" ("State(s) if False (\"\")")) -> ("States Out"=w421:string)  [unwired: 12 in]
        n160 = call <vilib>:"Add State(s) to Queue__jki_lib_state_machine.vi"("State(s) in Front (\"\")"=w421, "State(s) in (\"\")"=w430) -> ("States Out"=w429:string)  [unwired: 13 in]
      }
      frame "eSTOP1 Test: Start Timer (Start)" {
        # "Template Separator\n(You can make a copy of, or modify, this frame)"
        n161 = call "Timer.vi"("error in (no error)"=w433, "Enum"=T4."Start Timer") -> ("error out"=w437:errorcluster)  [unwired: 6 in, 3 out]
        n162 = property on="Timeout - Error Test" class="Slide (strict)"(error in=w437, "Value"=0.0 ("Horizontal Pointer Slide"), "Scale.Maximum"=3.0 ("Target Time"), "Scale.Minimum"=0.0 ("Scale.Range:Minimum")) -> (error out=w432:errorcluster)  [unwired: 1 in, 1 out]
        n163 = call <vilib>:"Add State(s) to Queue__jki_lib_state_machine.vi"("State(s) in Front (\"\")"="" ("State(s) if True (\"\")"), "State(s) in (\"\")"=w441) -> ("States Out"=w440:string)  [unwired: 13 in]
      }
      frame "eSTOP1 Test: Start Command (Error)" {
        # "Data"
        # "Length"
        # "ID"
        # "Target"
        # "Type"
        # "Pkt ID"
        # "Measurement initialisation code goes here"
        n164 = Unbundle By Name(w459) -> ("connection ID"=w457:refnum<k16>)
        n165 = Build Array(u8 91 ("element"), u8 1 ("element"), u8 9 ("element"), u8 110 ("element"), u8 0 ("element")) -> (w451:u8[])
        n166 = String To IP(1:"192.168.201.21" ("name")) -> (0:w455:u32)
        n167 = Byte Array To String(unsigned byte array=w451) -> (string=w445:string)
        n168 = UDP Write(address=w455, port or service name=u16 54321, connection ID=w457, data in=w445, 8:w458, 9:1000 ("timeout ms (25000)")) -> (error out=w444:errorcluster, 3:w456:refnum<k16>)
        n169 = Bundle By Name(cluster=w459, "connection ID"=w456) -> (w460:T5)
        n170 = call <userlib>:"Wait (ms)__ogtk.vi"("error in (no error)"=w444, "milliseconds to wait"=u32 5000) -> ("error out"=w443:errorcluster)  [unwired: 8 in, 1 out]
        n171 = call <vilib>:"Add State(s) to Queue__jki_lib_state_machine.vi"("State(s) in (\"\")"=w462) -> ("States Out"=w461:string)  [unwired: 14 in]
      }
      frame "eSTOP1 Test: Elapsed Timer (Start)" {
        # "check if timer elapsed if true end of test if false UDP is read again,"
        # "Template Separator\n(You can make a copy of, or modify, this frame)"
        n172 = call "Timer.vi"("error in (no error)"=w467, "Target Time"=3.0, "Enum"=T4."Get Time") -> ("error out"=w466:errorcluster, "Time Elapsed?"=w468:bool, "Elapsed Time"=→"Timeout - Error Test 2":dbl)  [unwired: 5 in, 1 out]
        n173 = call-poly <vilib>:"Select State(s)__jki_lib_state_machine.vi"("State(s) if True (\"\")"="Macro: Limits" ("State(s) if True (\"\")"), "Select"=w468, "State(s) if False (\"\")"="" ("State(s) if False (\"\")")) -> ("States Out"=w465:string)  [unwired: 12 in]
        n174 = call <vilib>:"Add State(s) to Queue__jki_lib_state_machine.vi"("State(s) in Front (\"\")"=w465, "State(s) in (\"\")"=w474) -> ("States Out"=w473:string)  [unwired: 13 in]
      }
    }
    n175 = Wait (ms)(milliseconds to wait=u32 1) -> ()  [unwired: 1 out]
  }
  "error out" <- w1
